vi "Build Waveform Header.vi"(8 "error in (no error)":errorcluster, 11 "DAQ Task in":refnum<class "DAQ Task.lvclass">) -> (0 "error out":errorcluster, 2 "Wfm Header":T1, 3 "DAQ Task out":refnum<class "DAQ Task.lvclass">)   [LabVIEW 2018, in "Data Acquisition.lvlib" / "DAQ Task.lvclass"]
uses:
  DAQ Task.lvclass
  Common/Controls/Waveform Header.ctl
  DAQ Task.lvclass/DAQ Task.ctl
  Measurements/Class Channel/Read ChanName.vi
  Measurements/Class Channel/Read Unit_EU.vi
  Measurements/Class Channel/Channel.lvclass
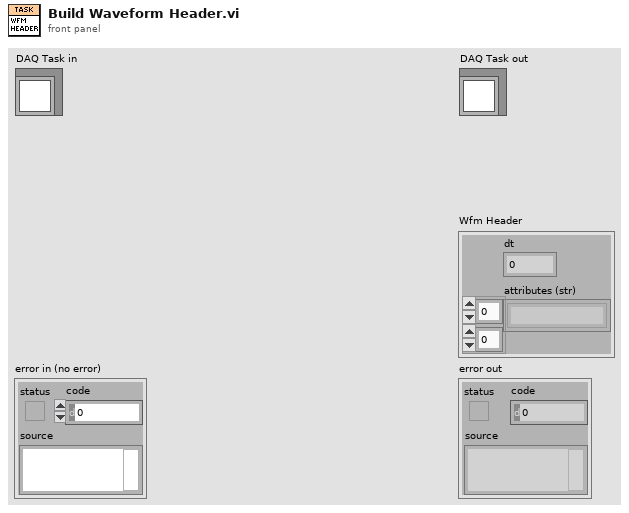
[diagram p1: front panel]
types:
  T1 = typedef "Waveform Header.ctl" = cluster{"dt":dbl, "attributes (str)":string[][]}
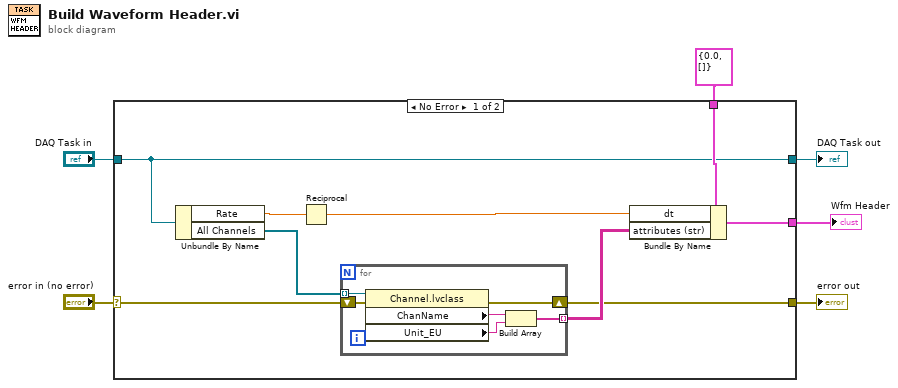
[diagram p0: block diagram]
diagram:
  n1 = case shown="No Error" "error in (no error)" {
    selector: "error in (no error)" -> [w9 w24]
    tunnel: [w7 w24] -> w5
    tunnel: [w13 w23] -> w3
    tunnel: "DAQ Task in" -> [w13 w23]
    tunnel: T1 {"dt"=0.0, "attributes (str)"=[]} ("Wfm Header") -> [w15 w22]
    tunnel: [w14 w22] -> w1
    frame No Error {
      n2 = Unbundle By Name(w13) -> ("Rate"=w12:dbl, "All Channels"=w10:refnum<class "Channel.lvclass">[])
      n3 = Reciprocal(x=w12) -> (1/x=w11:dbl)
      n4 = for {
        tunnel: w10 -> [w21] mode=indexing
        shift-right: [w19] -> w7
        shift-left: w9 -> [w20]
        tunnel: [w16] -> w8 mode=indexing
        n5 = property class="Channel.lvclass"(reference=w21, error in=w20) -> (error out=w19:errorcluster, "ChanName"=w18:string, "Unit_EU"=w17:string)  [unwired: 1 out]
        n6 = Build Array(w18, w17) -> (w16:string[])
      }
      n7 = Bundle By Name(cluster=w15, "dt"=w11, "attributes (str)"=w8) -> (w14:T1)
    }
    frame Error {
    }
  }
  "error out" <- w5
  "DAQ Task out" <- w3
  "Wfm Header" <- w1
